vi "Gyro Report.vi"(8 "error in (no error)":errorcluster) -> ()   [LabVIEW 2017]
uses:
  <vilib>/Rock Robotics/WPI/ThirdParty/Sensors/navX/_TypeDefs/FRIC_navX_DeviceNumbersTypeDef.ctl
  <vilib>/Rock Robotics/Network Tables/NT Write Number.vi
  <vilib>/Rock Robotics/Network Tables/NT Write Boolean.vi
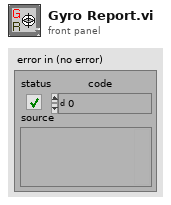
[diagram p1: front panel]
types:
  T1 = typedef "FRIC_navX_DeviceNumbersTypeDef.ctl" = enum16{"Dev0", "Dev1", "Dev2", "Dev3"}
  T2 = cluster{"Rollover":dbl, "Yaw":dbl, "Cont Yaw":dbl}
  T3 = typedef "WPI_EncoderDevRef.ctl" = cluster{"DevStatus":errorcluster, "EncoderIndex":T4, "CounterIndex":T5, "DistancePerCount":dbl, "Decoding Type":T6}
  T4 = typedef "FPGA_EncoderIdx.ctl" = enum8{"Enc 0", "Enc 1", "Enc 2", "Enc 3", "Enc 4", "Enc 5", "Enc 6", "Enc 7", "Invalid"}
  T5 = typedef "FPGA_CounterCtrSystemIndex.ctl" = enum8{"Ctr 0", "Ctr 1", "Ctr 2", "Ctr 3", "Ctr 4", "Ctr 5", "Ctr 6", "Ctr 7", "Invalid"}
  T6 = typedef "WPI_EncoderType.ctl" = enum16{"1x", "2x", "4x"}
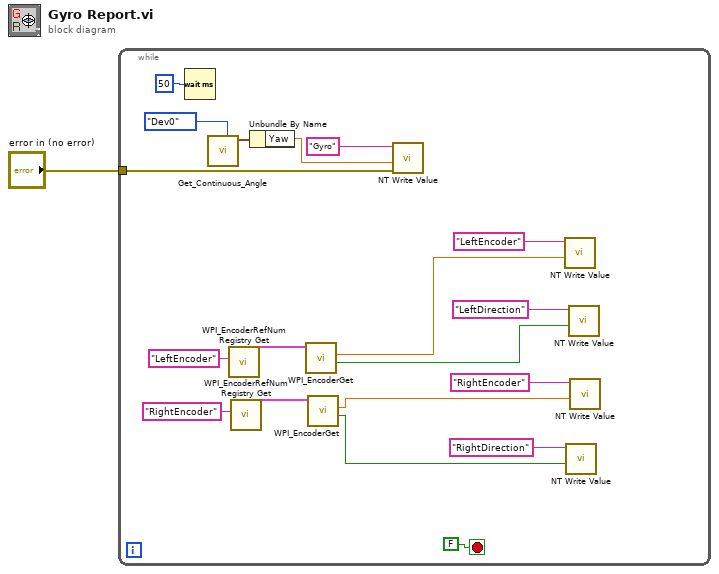
[diagram p0: block diagram]
diagram:
  n1 = while {
    tunnel: "error in (no error)" -> [w16]
    stop <- FALSE stop-if-true
    n2 = Wait (ms)(milliseconds to wait=u32 50) -> ()  [unwired: 1 out]
    n3 = call <vilib>:"Get_Continuous_Angle.vi"("Device Number"=FRIC_navX_DeviceNumbersTypeDef."Dev0") -> ("Continuous Angle"=w19:T2)  [unwired: 10 in]
    n4 = call <vilib>:"WPI_EncoderRefNum Registry Get.vi"("refnum name"="LeftEncoder") -> ("EncoderDevRef"=w11:T3)  [unwired: 9 in, 1 out]
    n5 = call <vilib>:"WPI_EncoderRefNum Registry Get.vi"("refnum name"="RightEncoder") -> ("EncoderDevRef"=w13:T3)  [unwired: 9 in, 1 out]
    n6 = Unbundle By Name(w19) -> ("Yaw"=w18:dbl)
    n7 = call <vilib>:"WPI_EncoderGet.vi"("EncoderDevRef"=w11) -> ("Direction"=w6:bool, "Distance"=w3:dbl)  [unwired: 5 in, 4 out]
    n8 = call <vilib>:"WPI_EncoderGet.vi"("EncoderDevRef"=w13) -> ("Direction"=w7:bool, "Distance"=w5:dbl)  [unwired: 5 in, 4 out]
    n9 = call-poly <vilib>:"NT Write Value.vi"("error in"=w16, "Numeric"=w18, "Name"="Gyro") -> ()  [unwired: 8 in, 1 out]
    n10 = call-poly <vilib>:"NT Write Value.vi"("Numeric"=w3, "Name"="LeftEncoder") -> ()  [unwired: 9 in, 1 out]
    n11 = call-poly <vilib>:"NT Write Value.vi"("Boolean"=w7, "Name"="RightDirection") -> ()  [unwired: 9 in, 1 out]
    n12 = call-poly <vilib>:"NT Write Value.vi"("Boolean"=w6, "Name"="LeftDirection") -> ()  [unwired: 9 in, 1 out]
    n13 = call-poly <vilib>:"NT Write Value.vi"("Numeric"=w5, "Name"="RightEncoder") -> ()  [unwired: 9 in, 1 out]
  }
